vi "Main.vi"() -> ()   [LabVIEW 2024]
doc: "Event-driven Queue State Machine (EDQSM) template in LabVIEW, designed to manage states and data via a queue. It includes three subVIs to create, enqueue, and dequeue states with attached data (using Variant for flexibility). The functional example features a simple interface with buttons that trigger events. The template is easily transformable into a traditional Queue State Machine (QSM) by removing the Wait state.\n\n<b>Disclaimer</b>: On the Use of the Term \"State Machine\"\nThis example is presented as an Event-Driven Queued State Machine (EDQSM), accurately describing its structure and behavior: states (or tasks) are managed via a queue and executed within an event-driven loop.\n\nHowever, it is important to note that in the LabVIEW development community, it is widely discussed that this kind of architecture —commonly found in QMH, DQMH, and similar designs— does not represent a formal State Machine in the strict sense, because the execution flow is not determined solely by internal state-transition logic, but may be affected by multiple external sources enqueueing messages asynchronously (external enqueueing).\n\nIn a deterministic State Machine, the system is always in one well-defined state, and transitions to the next state are determined exclusively by the current state and internal conditions, without interference from outside sources. When external actors (such as UI events, timers, or parallel modules) can insert messages into the queue at arbitrary times, this determinism is lost.\n\nFor this reason, many experienced developers recommend not referring to a Message Handler Loop (MHL) as a State Machine, since that distinction is crucial for avoiding design flaws, unpredictable behaviors, and debugging difficulties.\n\nThat said, this template supports a flexible structure that can behave deterministically if access to the queue is tightly controlled, or it can be extended as a more dynamic task handler system. The design choice depends on the specific goals of the application, but understanding the implications is essential for robust architecture."
uses:
  <vilib>/ErrorRing/Error Ring.xnode
  Event-Driven QSM/ED Queued State Machine.lvlib
  Event-Driven QSM/data--cluster.ctl
  Event-Driven QSM/queue state & data (Array).vi
  Event-Driven QSM/queue state & data (Single).vi
  <vilib>/Utility/error.llb/Error Cluster From Error Code.vi
panel:
  in  "Run Test 2":bool
  in  "Run Test 1":bool
  in  "Stop Button":bool
  # "EV Queued State Machine (State & Data)"
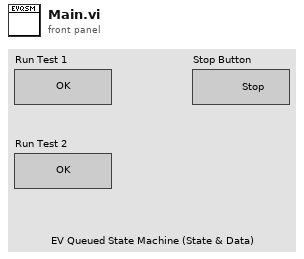
[diagram p1: front panel]
types:
  T1 = typedef "ED Queued State Machine.lvlib/data--cluster.ctl" = cluster{"Boolean":bool, "String":string, "Numeric":dbl, "Run Test1 Ref":refnum<vi>, "Run Test2 Ref":refnum<vi>, "Stop Butt Ref":refnum<vi>}
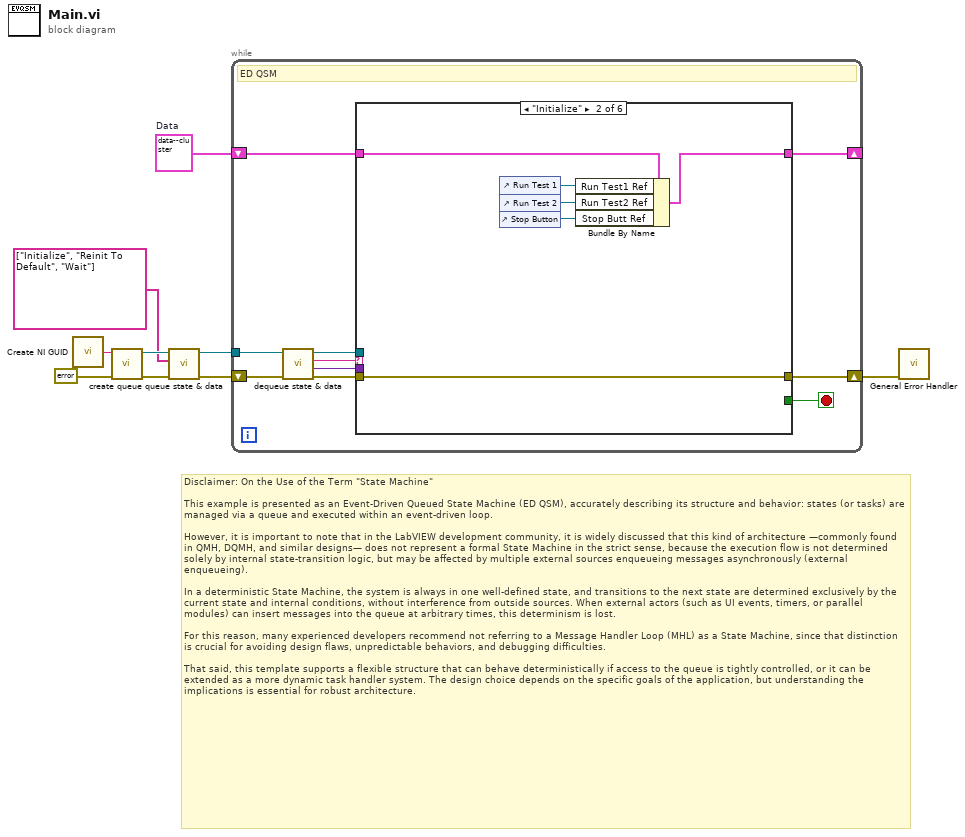
[diagram p0: block diagram]
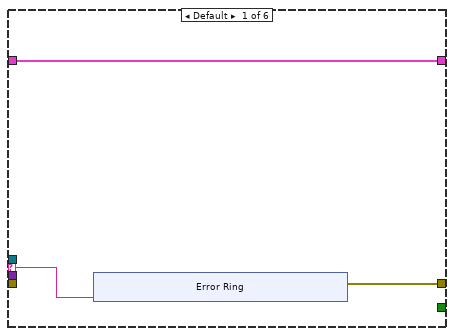
[diagram p2: hidden frame]
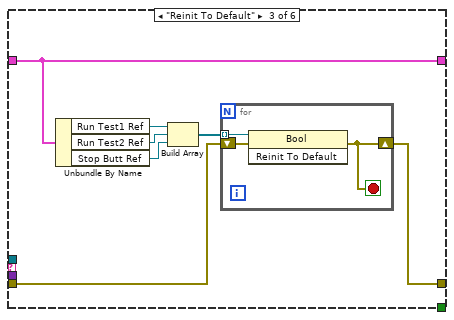
[diagram p3: hidden frame]
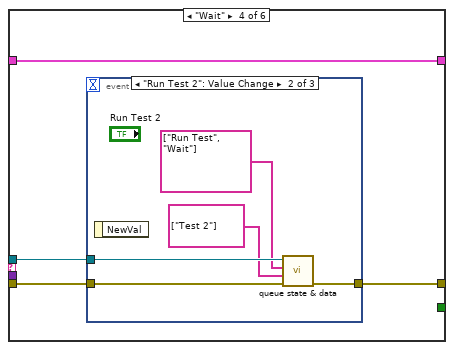
[diagram p4: hidden frame]
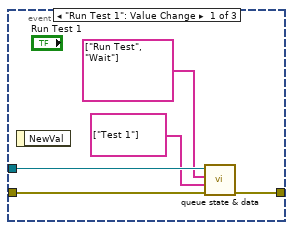
[diagram p5: hidden frame]
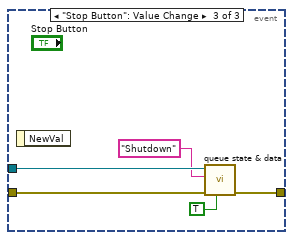
[diagram p6: hidden frame]
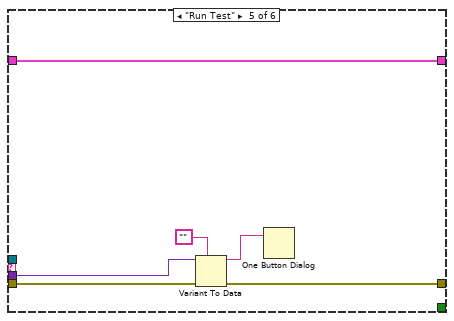
[diagram p7: hidden frame]
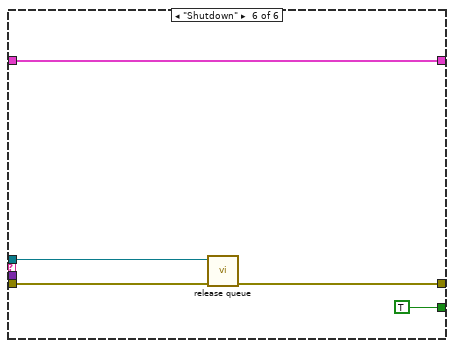
[diagram p8: hidden frame]
diagram:
  w4 = T1 {"Boolean"=FALSE, "String"="", "Numeric"=0.0, "Run Test1 Ref"=refnum, "Run Test2 Ref"=refnum, "Stop Butt Ref"=refnum}  # Data
  # "Disclaimer: On the Use of the Term \"State Machine\"\n\nThis example is presented as an Event-Driven Queued State Machine (ED QSM), accurately describing its structure and behavior: states (or tasks) are managed via a queue and executed within an event-driven loop.\n\nHowever, it is important to note that in the LabVIEW development community, it is widely discussed that this kind of architecture —commonly found in QMH, DQMH, and similar designs— does not represent a formal State Machine in the strict sense, because the execution flow is not determined solely by internal state-transition logic, but may be affected by multiple external sources enqueueing messages asynchronously (external enqueueing).\n\nIn a deterministic State Machine, the system is always in one well-defined state, and transitions to the next state are determined exclusively by the current state and internal conditions, without interference from outside sources. When external actors (such as UI events, timers, or parallel modules) can insert messages into the queue at arbitrary times, this determinism is lost.\n\nFor this reason, many experienced developers recommend not referring to a Message Handler Loop (MHL) as a State Machine, since that distinction is crucial for avoiding design flaws, unpredictable behaviors, and debugging difficulties.\n\nThat said, this template supports a flexible structure that can behave deterministically if access to the queue is tightly controlled, or it can be extended as a more dynamic task handler system. The design choice depends on the specific goals of the application, but understanding the implications is essential for robust architecture."
  n1 = call <vilib>:"Create NI GUID.vi"() -> ("NI GUID"=w1:string)
  n2 = call "create queue.vi"("error in (no error)"=errorcluster {"status"=FALSE, "code"=0, "source"=""} ("error constant"), "name (unnamed)"=w1) -> ("error out"=w6:errorcluster, "queue out"=w8:refnum<queue>)  [unwired: 7 in, 1 out]
  n3 = call-poly "queue state & data.vi"("error in (no error)"=w6, "State Array"=string[] ["Initialize", "Reinit To Default", "Wait"], "queue in"=w8) -> ("error out"=w7:errorcluster, "queue out"=w5:refnum<queue>)  [unwired: 7 in]
  n4 = while {
    shift-right: [w19] -> w9
    shift-left: w7 -> [w14]
    tunnel: w5 -> [w12]
    shift-right: [w10] -> _
    shift-left: w4 -> [w11]
    stop <- w18 stop-if-true
    # "ED QSM"
    n5 = call "dequeue state & data.vi"("error in (no error)"=w14, "queue in"=w12) -> ("error out"=w17:errorcluster, "State Data"=w15:variant, "State"=w16:string, "queue out"=w13:refnum<queue>)  [unwired: 6 in]
    n6 = case shown="\"Initialize\"" w16 {
      selector: w16 -> [w21 _ _ _ _ _]
      tunnel: w17 -> [_ w30 w37 w49 w70 w74]
      tunnel: [w22 w30 w36 w48 w69 w72] -> w19
      tunnel: [_ _ _ _ _ TRUE] -> w18
      tunnel: w13 -> [_ _ _ w47 _ w73]
      tunnel: w15 -> [_ _ _ _ w68 _]
      tunnel: w11 -> [w20 w35 w42 w46 w65 w71]
      tunnel: [w20 w34 w42 w46 w65 w71] -> w10
      frame Default {
        n7 = xnode ("Error Ring")("parameter 0"=w21) -> ("error out"=w22:errorcluster)
      }
      frame "Initialize" {
        n8 = control-ref of="Run Test 1"() -> (w33:refnum<vi>)
        n9 = control-ref of="Run Test 2"() -> (w32:refnum<vi>)
        n10 = control-ref of="Stop Button"() -> (w31:refnum<vi>)
        n11 = Bundle By Name(cluster=w35, "Run Test1 Ref"=w33, "Run Test2 Ref"=w32, "Stop Butt Ref"=w31) -> (w34:T1)
      }
      frame "Reinit To Default" {
        n12 = Unbundle By Name(w42) -> ("Run Test1 Ref"=w41:refnum<vi>, "Run Test2 Ref"=w40:refnum<vi>, "Stop Butt Ref"=w39:refnum<vi>)
        n13 = Build Array(w41, w40, w39) -> (w38:refnum<vi>[])
        n14 = for {
          tunnel: w38 -> [w45] mode=indexing
          shift-right: [w43] -> w36
          shift-left: w37 -> [w44]
          stop <- w43 stop-if-true
          n15 = invoke on="Invoke Node" class="Bool" method="Reinit To Default"(reference=w45, error in=w44) -> (error out=w43:errorcluster)  [unwired: 1 in, 2 out]
        }
      }
      frame "Wait" {
        n16 = event shown="[1] \"Run Test 2\": Value Change" {
          selector: _ -> [_ _ _]
          dyn-events: _ -> [_ _ _]
          timeout: _ -> [_ _ _]
          tunnel: w49 -> [w54 w59 w63]
          tunnel: [w53 w58 w64] -> w48
          tunnel: w47 -> [w52 w57 w62]
          event "Run Test 1": Value Change {
            n17 = event-data() -> ()  [unwired: 1 in, 1 out]
            n18 = call-poly "queue state & data.vi"("error in (no error)"=w54, "State Data Array"=string[] ["Test 1"], "State Array"=string[] ["Run Test", "Wait"], "queue in"=w52) -> ("error out"=w53:errorcluster)  [unwired: 6 in, 1 out]
          }
          event "Run Test 2": Value Change {
            n19 = event-data() -> ()  [unwired: 1 in, 1 out]
            n20 = call-poly "queue state & data.vi"("error in (no error)"=w59, "State Data Array"=string[] ["Test 2"], "State Array"=string[] ["Run Test", "Wait"], "queue in"=w57) -> ("error out"=w58:errorcluster)  [unwired: 6 in, 1 out]
          }
          event "Stop Button": Value Change {
            n21 = event-data() -> ()  [unwired: 1 in, 1 out]
            n22 = call-poly "queue state & data.vi"("Priority State? (F)"=TRUE ("Priority? (F)"), "error in (no error)"=w63, "State"="Shutdown", "queue in"=w62) -> ("error out"=w64:errorcluster)  [unwired: 6 in, 1 out]
          }
        }
      }
      frame "Run Test" {
        n23 = Variant To Data(error in=w70, type="" ("Empty String Constant"), Variant=w68) -> (data=w66:string, error out=w69:errorcluster)
        n24 = One Button Dialog(message=w66) -> ()  [unwired: 1 in, 1 out]
      }
      frame "Shutdown" {
        n25 = call "release queue.vi"("error in (no error)"=w74, "Queue in"=w73) -> ("error out"=w72:errorcluster)  [unwired: 9 in]
      }
    }
  }
  n26 = call <vilib>:"General Error Handler.vi"("error in (no error)"=w9) -> ()  [unwired: 10 in, 5 out]
